vi "LEBITplc.SetMon.vi"(0 "index of element":i32, 3 "i attribute in":T4, 5 "Data":dbl) -> ()   [LabVIEW 2014, in "LEBITplc.lvlib"]
uses:
  LEBITplc.lvlib
  CS_Core/CSSystem/CoreDefs/CoreDefs.call_type.ctl
  CS_Core/BaseProcess/BaseProcess.descriptor string definition.ctl
  CS_Core/CSSystem/CoreDefs/CoreDefs.rawDataType.ctl
  LEBITplc.i attribute.ctl
  CS_Core/CSSystem/CoreLib/CoreLib.string 2 byte array.vi
  CS_Core/CSSystem/CoreLib/CoreLib.double 2 byte array.vi
  CS_Core/CSSystem/CoreLib/CoreLib.short 2 byte array.vi
  CS_Core/CSSystem/CoreLib/CoreLib.lvlib
  CS_Core/BaseProcess/BaseProcess.lvlib
panel:
  out "error out":errorcluster
  out "call cluster out":T1={"Object"="", "Selector"="", "CallType"=enum."synchronous", "Async Object"="", "Async Selector"="", "Data Descriptor"="", "Data"=[], "Error #"=0, "Expire"=0}
  out "monValuePLC":string
  in  "call cluster in":T1={"Object"="", "Selector"="", "CallType"=enum."synchronous", "Async Object"="", "Async Selector"="", "Data Descriptor"="", "Data"=[], "Error #"=0, "Expire"=0}
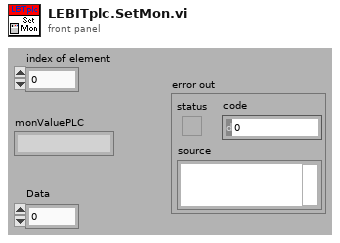
[diagram p1: front panel]
types:
  T1 = typedef "CoreDefs.call_type.ctl" = cluster{"Object":string, "Selector":string, "CallType":enum16{"simple", "synchronous", "asynchronous"}, "Async Object":string, "Async Selector":string, "Data Descriptor":T2, "Data":T3, "Error #":i32, "Expire":u32}
  T2 = typedef "BaseProcess.lvlib/BaseProcess.descriptor string definition.ctl" = string
  T3 = typedef "CoreDefs.rawDataType.ctl" = i8[]
  T4 = typedef "LEBITplc.lvlib/LEBITplc.i attribute.ctl" = cluster{"LLFLocation":string, "SetFileLocation":string, "nickNames":string[], "setValuePLCServiceID":i32[], "GUIServiceID":i32[], "monValuePLC":string[], "SetValueServiceID":i32[], "MonValueServiceID":i32[], "SetValue":dbl[][], "SetValueMin":dbl[], "SetValueMax":dbl[], "SetValueInfoServiceID":i32[], "GUINames":string[], "ListOfBases":string[], "Scale":dbl[], "Offset":dbl[], "setValuePLC":string[], "BaseName":string[], "ScaleServiceID":i32[], "OffsetServiceID":i32[], "AllPLCValues":string[], "CondSpecialArray":string[][], "CondSpecialIndex":i32[], "CondSpecialMonValue":dbl[], "RecentlyChanged":i32[], "SetFileLocationID":i32, "Dependent-Monitors":string[][], "LastLoadedFiles":string[], "IonGuideCalibLocation":string, "Monitor Dependent":string[], "Special":string[], "PLC?":bool[], "Start Date":string, "ListOfBasesServiceID":i32, "SETRA VISA resource":refnum<visa-resource-name>}
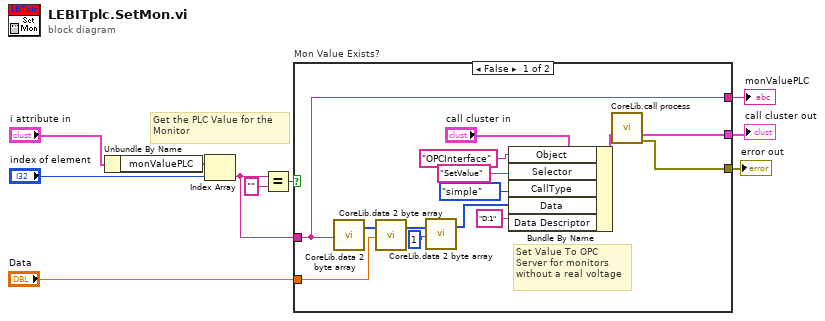
[diagram p0: block diagram]
diagram:
  # "Get the PLC Value for the \nMonitor"
  n1 = Unbundle By Name("i attribute in") -> ("monValuePLC"=w9:string[])
  n2 = Index Array(array=w9, index="index of element") -> (element=w7:string)
  n3 = Equal?(x=w7, y="") -> (x = y?=w4:bool)
  n4 = case "Mon Value Exists?" shown="False" w4 {
    tunnel: w7 -> [w20 w25]
    tunnel: [w20 w25] -> w6
    tunnel: "Data" -> [w18 _]
    tunnel: [w16 _] -> w2
    tunnel: [w14 _] -> w1
    frame False {
      # "Set Value To OPC  \nServer for monitors\nwithout a real voltage"
      n5 = call-poly "CoreLib.data 2 byte array.vi"("string"=w20) -> ("byteArray out"=w19:T3)  [unwired: 18 in]
      n6 = call-poly "CoreLib.data 2 byte array.vi"("byteArray"=w19, "f64"=w18) -> ("byteArray out"=w13:T3)  [unwired: 17 in]
      n7 = call-poly "CoreLib.data 2 byte array.vi"("byteArray"=w13, "i16"=i16 1) -> ("byteArray out"=w12:T3)  [unwired: 17 in]
      n8 = Bundle By Name(cluster="call cluster in", "Object"="OPCInterface", "Selector"="SetValue" ("string"), "CallType"=enum16{"simple", "synchronous", "asynchronous"}."simple", "Data"=w12, "Data Descriptor"=T2 "D:1") -> (w17:T1)
      n9 = call "CoreLib.call process.vi"("call cluster in"=w17) -> ("call cluster out"=w14:T1, "error out"=w16:errorcluster)  [unwired: 13 in]
    }
    frame True {
    }
  }
  "monValuePLC" <- w6
  "error out" <- w2
  "call cluster out" <- w1
